vi "Get Redirects.vi"(0 "client handle":T1, 5 "url":string, 11 "error in (no error)":errorcluster, 12 "timeout (10000)":i32=10000, 13 "max redirects (21)":i32=21) -> (3 "headers":string, 4 "client handle out":T1, 6 "url out":string, 8 "num redirects":i32, 10 "redirected?":bool, 14 "redirect breadcrumb":string[](array[string]), 15 "error out":errorcluster)   [LabVIEW 2019, in "HTTP Client Extensions.lvlib"]
uses:
  HTTP Client Extensions.lvlib
  <vilib>/httpClient/ClientHandle.ctl
  <vilib>/httpClient/LabVIEWHTTPClient.lvlib
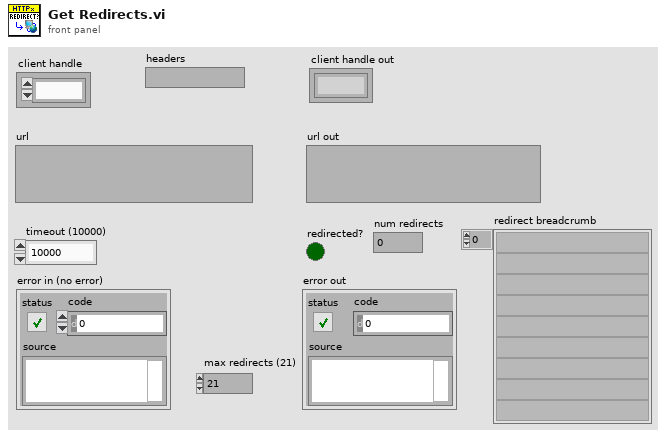
[diagram p1: front panel]
types:
  T1 = typedef "LabVIEWHTTPClient.lvlib/ClientHandle.ctl" = refnum<k1>
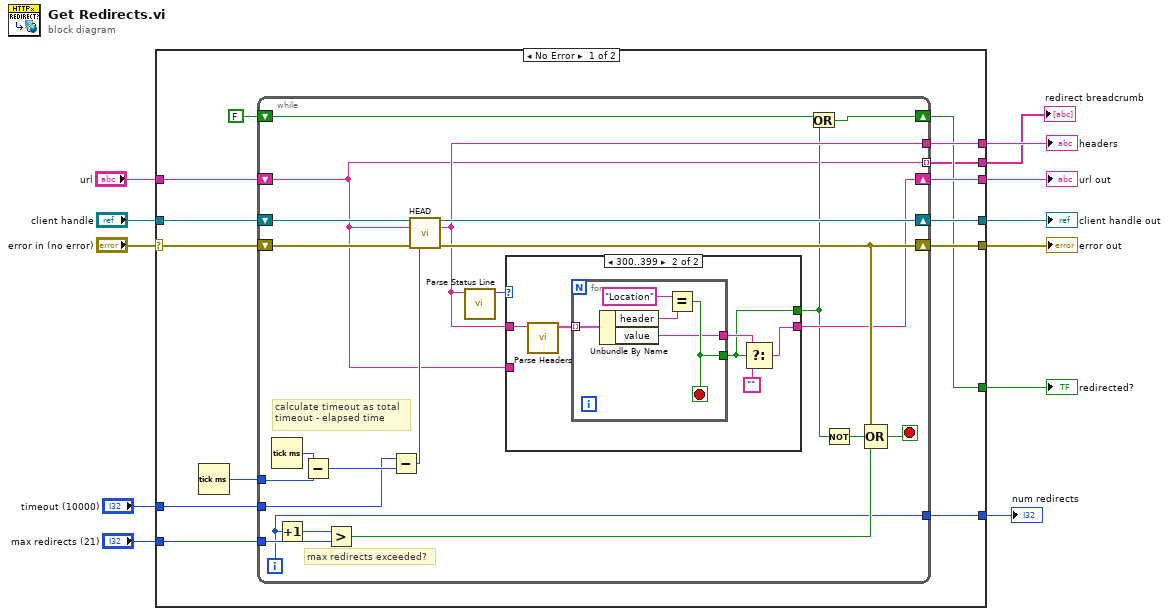
[diagram p0: block diagram]
diagram:
  n1 = case shown="No Error" "error in (no error)" {
    selector: "error in (no error)" -> [w22 w61]
    tunnel: "url" -> [w26 w63]
    tunnel: [w25 w62] -> w11
    tunnel: "client handle" -> [w24 w62]
    tunnel: [w23 w61] -> w9
    tunnel: [w21 _] -> w7
    tunnel: [w20 w63] -> w6
    tunnel: [w15 _] -> w5
    tunnel: "max redirects (21)" -> [w18 _]
    tunnel: "timeout (10000)" -> [w17 _]
    tunnel: [w14 _] -> w2
    tunnel: [w13 _] -> w1
    frame No Error {
      n2 = Tick Count (ms)() -> (millisecond timer value=w16:u32)
      n3 = while {
        shift-right: [w40] -> w20
        shift-left: w26 -> [w27]
        shift-right: [w47] -> w25
        shift-left: w24 -> [w46]
        shift-right: [w44] -> w23
        shift-left: w22 -> [w45]
        tunnel: [w41] -> w21
        shift-right: [w39] -> w15
        shift-left: FALSE -> [w37]
        tunnel: w18 -> [w36]
        tunnel: w17 -> [w30]
        tunnel: w16 -> [w33]
        tunnel: [w28] -> w14
        tunnel: [w27] -> w13 mode=indexing
        i -> [w28]
        stop <- w42 stop-if-true
        # "max redirects exceeded?"
        # "calculate timeout as total timeout - elapsed time"
        n4 = Tick Count (ms)() -> (millisecond timer value=w34:u32)
        n5 = Increment(x=w28) -> (x+1=w29:i32)
        n6 = Subtract(x=w34, y=w33) -> (x-y=w32:u32)
        n7 = Greater?(x=w29, y=w36) -> (0:w35:bool)
        n8 = Subtract(x=w30, y=w32) -> (x-y=w31:u32)
        n9 = call <vilib>:"HEAD.vi"("client handle"=w46, "url"=w27, "error in (no error)"=w45, "timeout (10000)"=w31) -> ("client handle out"=w47:T1, "headers"=w41:string, "error out"=w44:errorcluster)  [unwired: 9 in]
        n10 = call "Parse Status Line.vi"("Headers w/ status line"=w41) -> ("Status Code"=w48:u16)  [unwired: 6 in, 4 out]
        n11 = case shown="300..399" w48 {
          tunnel: w41 -> [_ w55]
          tunnel: [w49 w51] -> w40
          tunnel: [_ w50] -> w38
          tunnel: w27 -> [w49 _]
          frame Default {
          }
          frame 300..399 {
            n12 = call "Parse Headers.vi"("HTTP Headers"=w55) -> ("Response Headers"=w54:cluster{"header":string, "value":string}[])  [unwired: 10 in]
            n13 = for {
              tunnel: w54 -> [w60] mode=indexing
              tunnel: [w57] -> w50
              tunnel: [w56] -> w53
              stop <- w57 stop-if-true
              n14 = Unbundle By Name(w60) -> ("header"=w59:string, "value"=w56:string)
              n15 = Equal?(x="Location" ("header"), y=w59) -> (x = y?=w57:bool)
            }
            n16 = Select(t=w53, s=w50, f="") -> (s? t:f=w51:string)
          }
        }
        n17 = Or(x=w37, y=w38) -> (x .or. y?=w39:bool)
        n18 = Not(x=w38) -> (.not. x?=w43:bool)
        n19 = Compound Arithmetic op=OR(w44, w43, w35) -> (w42:bool)
      }
    }
    frame Error {
    }
  }
  "redirected?" <- w5
  "url out" <- w6
  "headers" <- w7
  "client handle out" <- w11
  "error out" <- w9
  "num redirects" <- w2
  "redirect breadcrumb" <- w1
